vi "get&set kV&mA (str).vi"(6 "Get/Set? (Set)":bool=TRUE, 8 "error in (no error)":errorcluster, 9 "mA In":string, 10 "kV In":string, 11 "VGS_ScanInfo in":refnum<class "VGS_ScanInfo.lvclass">) -> (0 "error out":errorcluster, 1 "mA Out":string, 2 "kV Out":string, 3 "VGS_ScanInfo out":refnum<class "VGS_ScanInfo.lvclass">)   [LabVIEW 2022 SP3, in "LV_VGS.lvlib" / "VGS_ScanInfo.lvclass"]
uses:
  VGS_ScanInfo.lvclass
  VGS_ScanInfo.lvclass/VGS_ScanInfo.ctl
  C:/Users/Andrey/Documents/GitHub/LV_VGS/vgs_project.dll
  vgs_project.dll
panel:
  # "-Set\n-Get"
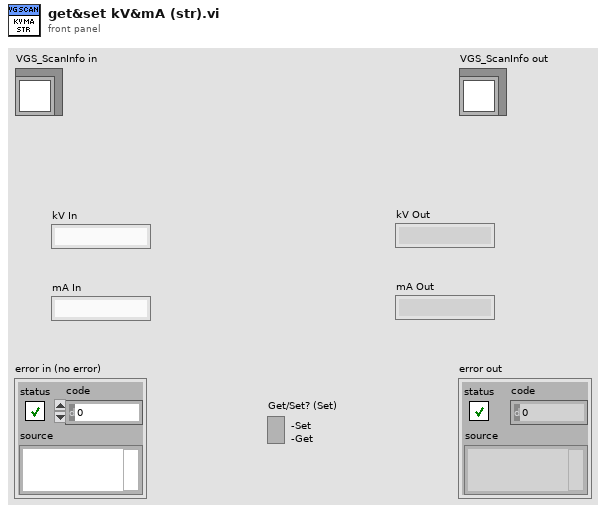
[diagram p1: front panel]
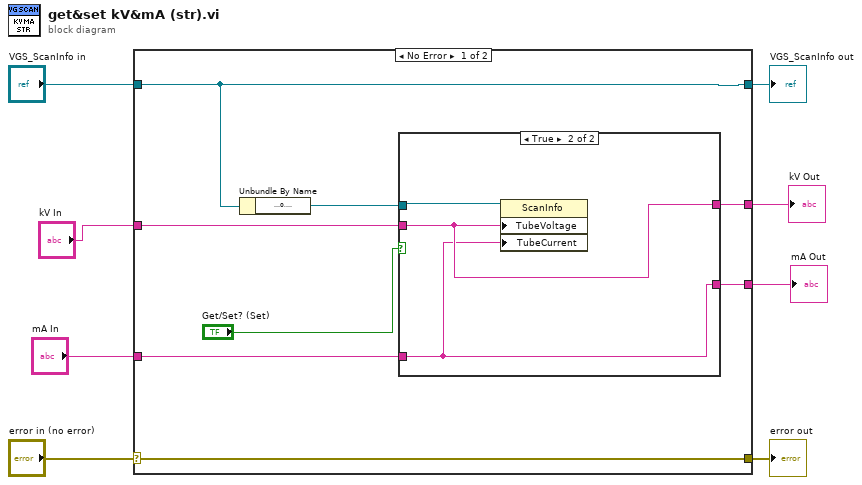
[diagram p0: block diagram]
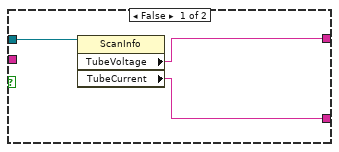
[diagram p2: hidden frame]
diagram:
  n1 = case shown="No Error" "error in (no error)" {
    selector: "error in (no error)" -> [w16 w25]
    tunnel: [w16 w25] -> w7
    tunnel: [w15 w26] -> w5
    tunnel: "VGS_ScanInfo in" -> [w15 w26]
    tunnel: [w12 w24] -> w4
    tunnel: [w11 w23] -> w3
    tunnel: "kV In" -> [w10 w24]
    tunnel: "mA In" -> [w9 w23]
    frame No Error {
      n2 = Unbundle By Name(w15) -> ("scan info"=w13:refnum<k24>)
      n3 = case shown="True" "Get/Set? (Set)" {
        tunnel: w13 -> [w19 w22]
        tunnel: [w18 w21] -> w12
        tunnel: [w17 w20] -> w11
        tunnel: w10 -> [_ w21]
        tunnel: w9 -> [_ w20]
        frame False {
          n4 = property class="ScanInfo"(reference=w19) -> ("TubeVoltage"=w18:string, "TubeCurrent"=w17:string)  [unwired: 1 in, 2 out]
        }
        frame True {
          n5 = property class="ScanInfo"(reference=w22, "TubeVoltage"=w21, "TubeCurrent"=w20) -> ()  [unwired: 1 in, 2 out]
        }
      }
    }
    frame Error {
    }
  }
  "error out" <- w7
  "VGS_ScanInfo out" <- w5
  "kV Out" <- w4
  "mA Out" <- w3
